vi "r12h.vi"() -> ()   [LabVIEW 2019]
panel:
  out "error out":errorcluster
  in  "error in (no error)":errorcluster
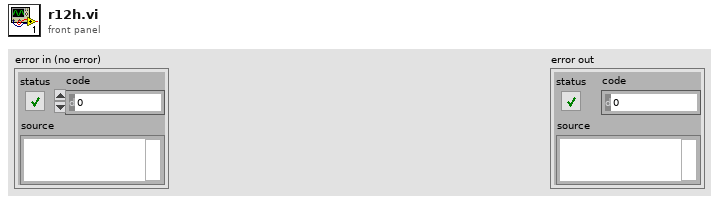
[diagram p1: front panel]
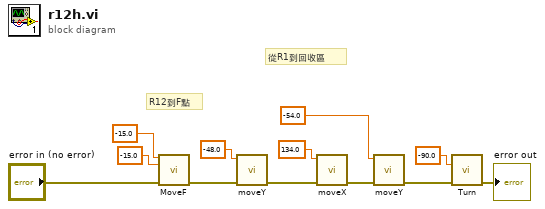
[diagram p0: block diagram]
diagram:
  # "R12到F點"
  # "從R1到回收區"
  n1 = call "MoveF.vi"("X"=-15.0, "Y"=-15.0, "error in (no error)"="error in (no error)") -> ("error out"=w1:errorcluster)  [unwired: 12 in]
  n2 = call "moveY.vi"("error in (no error)"=w1, "Y"=-48.0) -> ("error out"=w11:errorcluster)  [unwired: 9 in]
  n3 = call "moveX.vi"("error in (no error)"=w11, "X"=134.0) -> ("error out"=w9:errorcluster)  [unwired: 9 in]
  n4 = call "moveY.vi"("error in (no error)"=w9, "Y"=-54.0) -> ("error out"=w7:errorcluster)  [unwired: 9 in]
  n5 = call "Turn.vi"("角度"=-90.0, "error in (no error)"=w7) -> ("error out"=→"error out":errorcluster)  [unwired: 13 in]
